vi "sendEvt.vi"(8 "error in (no error)":errorcluster, 9 "Event Details":string="\"InPosition\" : true\n\n\"Tolerance\" : 0.2", 10 "Event Id":string="move", 11 "tcpServer in":refnum<class "TcpServer.lvclass">) -> (0 "error out":errorcluster, 3 "tcpServer out":refnum<class "TcpServer.lvclass">)   [LabVIEW 2018, in "TcpServer.lvclass"]
doc: "Send an event to the TCP Server to be read by the TCP Client."
uses:
  TcpServer.lvclass
  TcpServerCmd/typedef/eventTypeDef.ctl
  TcpServer.lvclass/TcpServer.ctl
  TcpServerCmd/TcpServerCmd.lvclass/TcpServerCmd.ctl
  TcpServerCmd/TcpServerCmd.lvclass
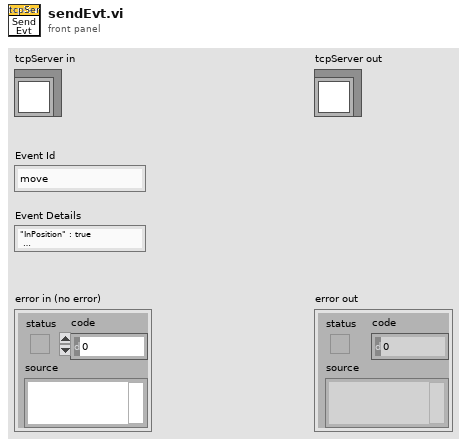
[diagram p1: front panel]
types:
  T1 = typedef "TcpServerCmd.lvclass/eventTypeDef.ctl" = cluster{"name":string, "evtDetails":string}
  T2 = typedef "TcpServerCmd.lvclass/userEventTypeDef.ctl" = cluster{"CmdRead":refnum<user-event>, "CmdWrite":refnum<user-event>, "EvtRead":refnum<user-event>, "EvtWrite":refnum<user-event>, "GenRead":refnum<user-event>, "GenWrite":refnum<user-event>}
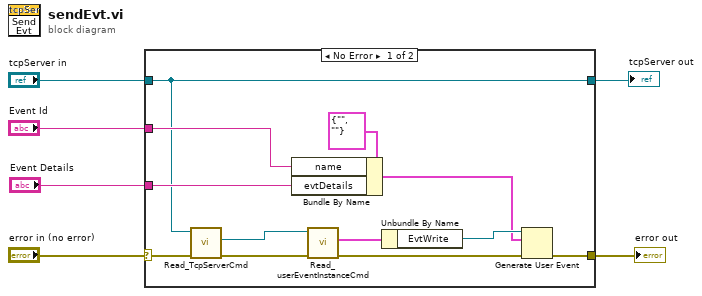
[diagram p0: block diagram]
diagram:
  n1 = case shown="No Error" "error in (no error)" {
    selector: "error in (no error)" -> [w10 w20]
    tunnel: [w17 w20] -> w5
    tunnel: "Event Details" -> [w18 _]
    tunnel: "Event Id" -> [w16 _]
    tunnel: "tcpServer in" -> [w7 w19]
    tunnel: [w7 w19] -> w1
    frame No Error {
      n2 = call "Read_TcpServerCmd.vi"("error in (no error)"=w10, "TcpServer in"=w7) -> ("error out"=w14:errorcluster, "TcpServerCmd.lvclass"=w15:refnum<class "TcpServerCmd.lvclass">)  [unwired: 7 in, 1 out]
      n3 = Bundle By Name(cluster=T1 {"name"="", "evtDetails"=""} ("Event"), "name"=w16, "evtDetails"=w18) -> (w11:T1)
      n4 = call "Read_userEventInstanceCmd.vi"("error in (no error)"=w14, "TcpServerCmd in"=w15) -> ("error out"=w9:errorcluster, "userEventInstance"=w13:T2)  [unwired: 7 in, 1 out]
      n5 = Unbundle By Name(w13) -> ("EvtWrite"=w12:refnum<user-event>)
      n6 = Generate User Event(user event=w12, event data cluster=w11, error in=w9) -> (error out=w17:errorcluster)  [unwired: 1 in, 1 out]
    }
    frame Error {
    }
  }
  "error out" <- w5
  "tcpServer out" <- w1
